vi "WeightedCrossMomentsWrapped.vi"(6 "Shift2In":T1[](array[typedef]), 8 "Shift1In":T2[](array[typedef]) {"Cross Correlation" format="%.2f"; "Stats" format="%.2f"}, 9 "IndicesIn":i32[][](array[numeric]), 10 "Time Trace in":T7[](array[typedef]), 11 "Analysis Info clusterIn":T4[](array[typedef]) {"Sync Delay Time (s)" format="%.4f"; "Total Meas Time (s)" format="%_5g"; "Sd Error in Variance" format="%_3g"; "Skew_u" format="%_3g"; "% u'/U" format="%_3g"; "Sd Error in Mean" format="%_3g"; "Kurt_u" format="%_3g"; "u^4" format="%_3g"; "u^3" format="%_3g"; "U" format="%_3g"; "u^2" format="%_3g"}) -> (0 "Shift1Out":T2[](array[typedef]) {"Cross Correlation" format="%.2f"; "Stats" format="%.2f"}, 2 "ResultsOut":T3[](array[typedef]) {"Time Window (ms)" format="%.2f"; "w^2 Paired" format="%.2f"; "u^2 Paired" format="%.2f"; "u^2w^2" format="%.2f"; "u^3w" format="%.2f"; "uw^3" format="%.2f"; "uw/u'w'" format="%.2f"; "uw^2" format="%.2f"; "u^2w" format="%.2f"; "uw" format="%.2f"}, 4 "Shift2Out":T1[](array[typedef]))   [LabVIEW 2021]
uses:
  Controls/Time_Trace_Cluster.ctl
  Controls/Analysis_info_cluster.ctl
  Controls/Inst_type.ctl
  Controls/Instrument_Array.ctl
  Controls/Correlation_cluster1.ctl
  Controls/Cross_Moments_Shift_Cluster.ctl
  Controls/Shift_Cluster.ctl
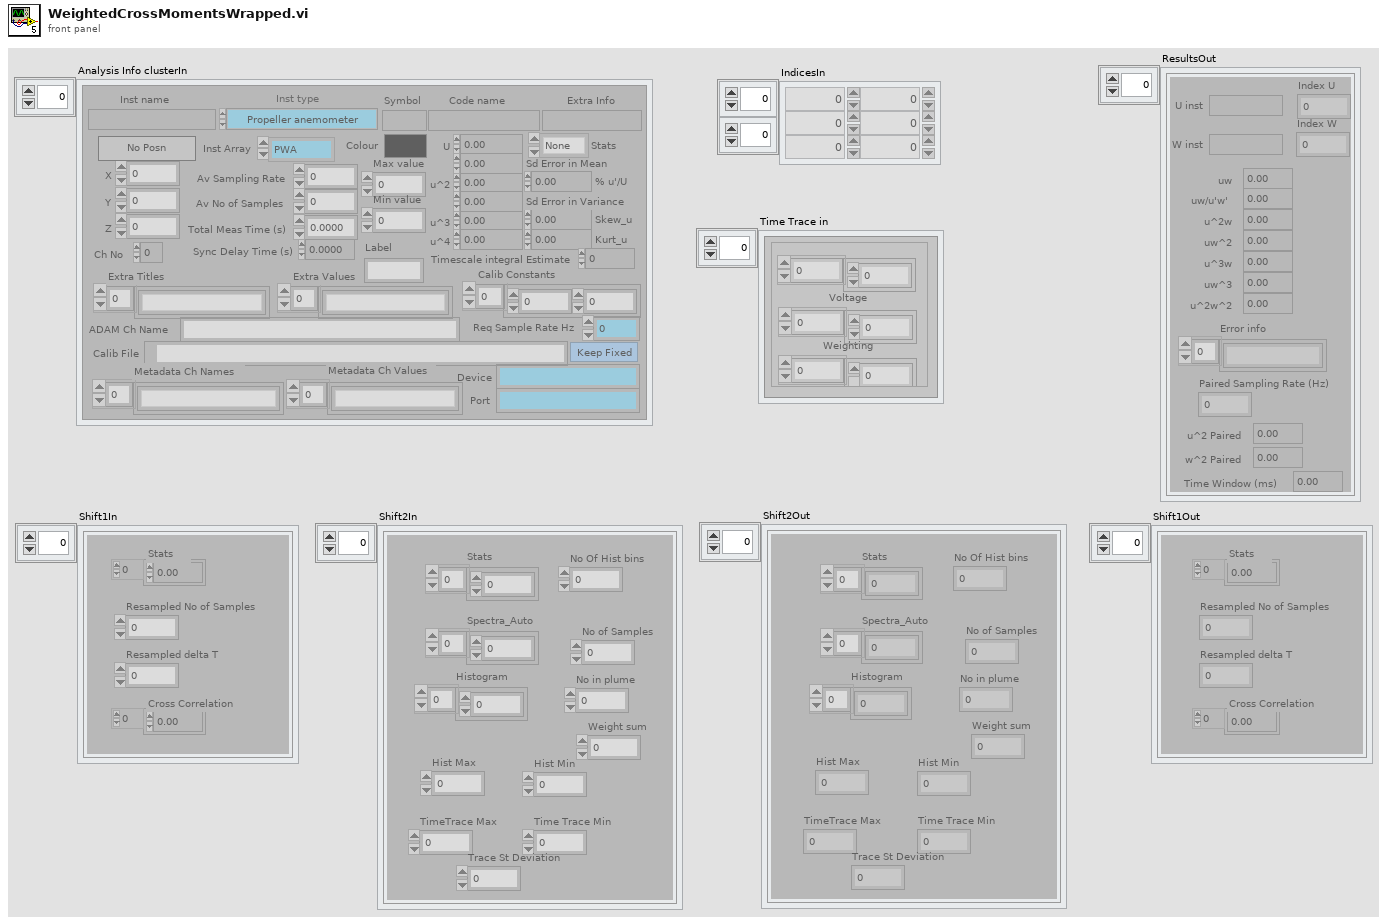
[diagram p1: front panel]
types:
  T1 = typedef "Shift_Cluster.ctl" = cluster{"Stats":dbl[], "Spectra_Auto":dbl[], "Histogram":dbl[], "Hist Max":dbl, "Hist Min":dbl, "No of Samples":i32, "No in plume":i32, "Weight sum":dbl, "No Of Hist bins":i32, "TimeTrace Max":dbl, "Time Trace Min":dbl, "Trace St Deviation":dbl}
  T2 = typedef "Cross_Moments_Shift_Cluster.ctl" = cluster{"Stats":dbl[], "Resampled No of Samples":i32, "Resampled delta T":dbl, "Cross Correlation":dbl[]}
  T3 = typedef "Correlation_cluster1.ctl" = cluster{"U inst":string, "uw":dbl, "u^2w":dbl, "uw^2":dbl, "uw/u'w'":dbl, "W inst":string, "uw^3":dbl, "u^3w":dbl, "u^2w^2":dbl, "Index U":i32, "Index W":i32, "Error info":string[], "Paired Sampling Rate (Hz)":dbl, "u^2 Paired":dbl, "w^2 Paired":dbl, "Time Window (ms)":dbl}
  T4 = typedef "Analysis_info_cluster.ctl" = cluster{"Colour":u32, "Inst type":T5, "Inst name":string, "Symbol":string, "Code name":string, "Extra Info":string, "Inst Array":T6, "Extra Titles":string[], "Extra Values":string[], "U":dbl, "u^2":dbl, "u^3":dbl, "u^4":dbl, "Skew_u":dbl, "Kurt_u":dbl, "Sd Error in Mean":dbl, "% u'/U":dbl, "X":dbl, "Y":dbl, "Z":dbl, "Timescale integral Estimate":dbl, "Sd Error in Variance":dbl, "Calib File":path, "Calib Constants":dbl[], "Output Position":bool, "Stats":enum16{"None", "Basic", "Full"}, "Av Sampling Rate":dbl, "Av No of Samples":dbl, "Total Meas Time (s)":dbl, "ADAM Ch Name":string, "Max value":dbl, "Min value":dbl, "Req Sample Rate Hz":dbl, "Sync Delay Time (s)":dbl, "Ch No":i16, "Device":string, "Use Latest Calib":bool, "Port":string, "Metadata Ch Names":string[], "Metadata Ch Values":string[], "Label":string}
  T5 = typedef "Inst_type.ctl" = enum16{"Raw voltage", "Raw with zero offsetting", "Propeller anemometer", "Pressure Transducer", "Pitot-static tube", "Hot wire", "Cross wire 1", "Cross wire 2", "Generic Linear", "Generic Polynomial", "Generic BackPoly", "Fast FID", "Thermocouple", "Cold wire", "Pulsed Wire", "LDA Vel", "LDA Tran time", "LDA Arr time", "Microphone"}
  T6 = typedef "Instrument_Array.ctl" = enum16{"PWA", "LDA", "Analogue"}
  T7 = typedef "Time_Trace_Cluster.ctl" = cluster{"Weighting":dbl[], "Voltage":dbl[], "Eng Values":dbl[]}
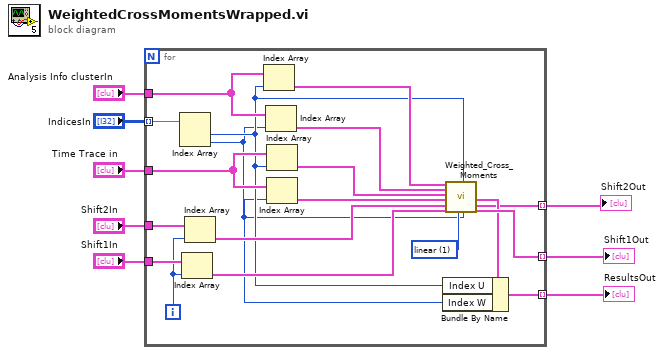
[diagram p0: block diagram]
diagram:
  n1 = for {
    tunnel: "IndicesIn" -> [w27] mode=indexing
    tunnel: "Analysis Info clusterIn" -> [w25]
    tunnel: [w23] -> w4 mode=indexing
    tunnel: "Shift1In" -> [w22]
    tunnel: [w19] -> w5 mode=indexing
    tunnel: "Time Trace in" -> [w18]
    tunnel: [w13] -> w2 mode=indexing
    tunnel: "Shift2In" -> [w12]
    i -> [w11]
    w15 = 1 items=["nearest", "linear", "spline", "cubic Hermite", "Lagrange"] ("interp. method")
    n2 = Index Array(array=w27) -> (element #1=w10:i32, element #2=w9:i32)  [unwired: 2 in]
    n3 = Index Array(array=w22, index=w11) -> (element=w21:T2)
    n4 = Index Array(array=w12, index=w11) -> (element=w14:T1)
    n5 = Index Array(array=w25, index=w10) -> (element=w26:T4)
    n6 = Index Array(array=w25, index=w9) -> (element=w24:T4)
    n7 = Index Array(array=w18, index=w10) -> (element=w17:T7)
    n8 = Index Array(array=w18, index=w9) -> (element=w16:T7)
    n9 = call "Weighted_Cross_Moments.vi"("AI Cluster 1"=w26, "AI Cluster 2"=w24, "Time Cluster 1"=w17, "Time Cluster 2"=w16, "Shift Cluster In"=w21, "Shift Input"=w14, "interp. method"=w15, "Index1"=w10, "Index2"=w9) -> ("Shift Output"=w13:T1, "output cluster"=w20:T3, "Shift Cluster Out"=w23:T2)  [unwired: 8 in]
    n10 = Bundle By Name(cluster=w20, "Index U"=w10, "Index W"=w9) -> (w19:T3)
  }
  "ResultsOut" <- w5
  "Shift1Out" <- w4
  "Shift2Out" <- w2
